vi "Store Data Core.vi"(8 "Error In":errorcluster, 10 "LHW-DataCollection":refnum<class "LHW-DataCollection.lvclass">, 11 "LHW-Storage-Actor in":refnum<class "LHW-Storage-Actor.lvclass">) -> (0 "Error Out":errorcluster, 3 "LHW-Storage-Actor out":refnum<class "LHW-Storage-Actor.lvclass">)   [LabVIEW 2016, in "LHW-Storage.lvlib" / "LHW-Storage-Actor.lvclass"]
doc: "Store received data."
uses:
  LHW-Storage-Actor.lvclass
  Classes/LHW-Data/LHW-DataCollection/LHW-DataCollection.lvclass
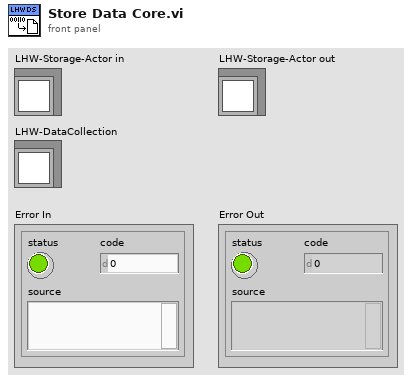
[diagram p1: front panel]
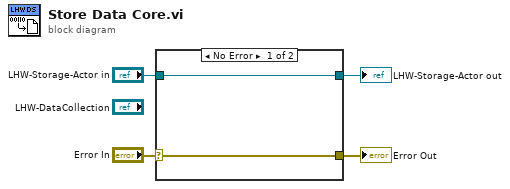
[diagram p0: block diagram]
diagram:
  n1 = case shown="No Error" "Error In" {
    selector: "Error In" -> [w5 w8]
    tunnel: [w5 w8] -> w3
    tunnel: [w6 w7] -> w1
    tunnel: "LHW-Storage-Actor in" -> [w6 w7]
    frame No Error {
    }
    frame Error {
    }
  }
  "Error Out" <- w3
  "LHW-Storage-Actor out" <- w1
